vi "Square Joystick.vi"(11 "In":dbl) -> (3 "Squared Output":dbl)   [LabVIEW 2018]
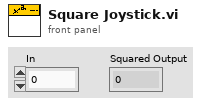
[diagram p1: front panel]
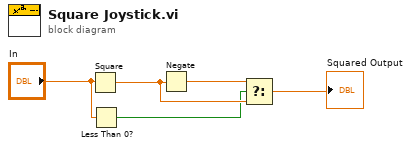
[diagram p0: block diagram]
diagram:
  n1 = Square(x="In") -> (x^2=w4:dbl)
  n2 = Less Than 0?(x="In") -> (x < 0?=w1:bool)
  n3 = Negate(x=w4) -> (-x=w2:dbl)
  n4 = Select(t=w2, s=w1, f=w4) -> (s? t:f=→"Squared Output":dbl)
